vi "Get SplitterPosition.vi"(8 "error in (no error)":errorcluster caption="错误输入（无错误）", 11 "PanelDataNode 输入":refnum<class "PanelDataNode.lvclass"> caption="DNL_LabVIEW Object in") -> (0 "error out":errorcluster caption="错误输出", 2 "SplitterPosition(relative)":dbl, 3 "PanelDataNode 输出":refnum<class "PanelDataNode.lvclass"> caption="DNL_LabVIEW Object out")   [LabVIEW 2016, in "PanelDataNode.lvclass"]
uses:
  PanelDataNode.lvclass
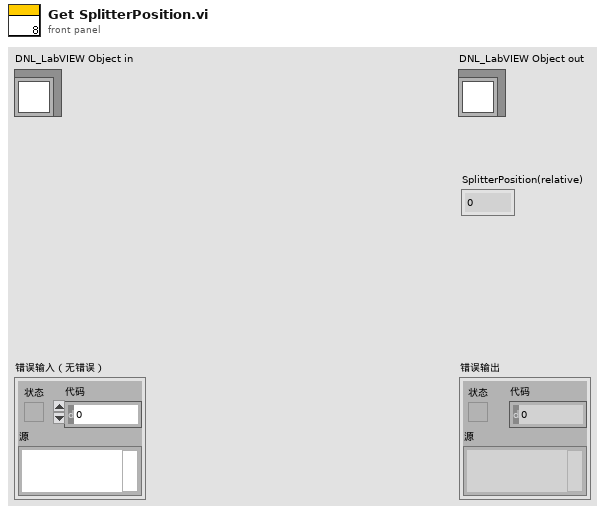
[diagram p1: front panel]
types:
  T1 = typedef "LVBoundsTypeDef.ctl" = cluster{"Width":u32, "Height":u32}
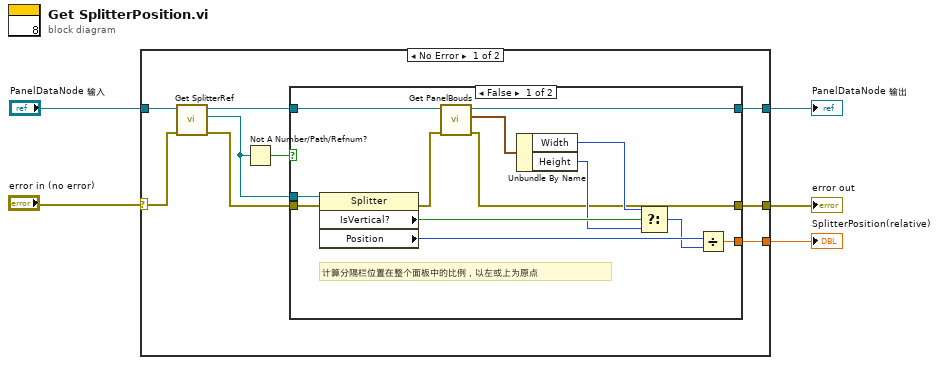
[diagram p0: block diagram]
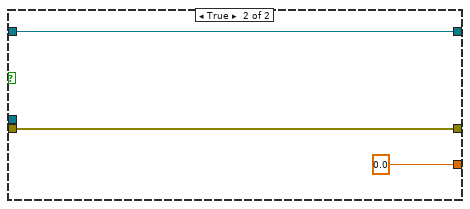
[diagram p2: hidden frame]
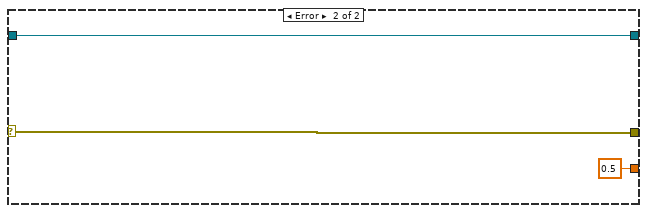
[diagram p3: hidden frame]
diagram:
  n1 = case shown="No Error" "error in (no error)" {
    selector: "error in (no error)" -> [w8 w33]
    tunnel: [w9 w33] -> w4
    tunnel: [w12 w32] -> w2
    tunnel: "PanelDataNode 输入" -> [w14 w32]
    tunnel: [w11 0.5] -> w1
    frame No Error {
      n2 = call "Get SplitterRef.vi"("error in"=w8, "PanelDataNode 输入"=w14) -> ("error out"=w10:errorcluster, "Splitter"=w7:refnum<vi>, "PanelDataNode 输出"=w13:refnum<class "PanelDataNode.lvclass">)  [unwired: 7 in]
      n3 = Not A Number/Path/Refnum?(number/path/refnum=w7) -> (NaN/Path/Refnum?=w6:bool)
      n4 = case shown="False" w6 {
        tunnel: w13 -> [w27 w29]
        tunnel: [w26 w29] -> w12
        tunnel: [w19 0.0] -> w11
        tunnel: w10 -> [w18 w28]
        tunnel: [w16 w28] -> w9
        tunnel: w7 -> [w15 _]
        frame False {
          # "计算分隔栏位置在整个面板中的比例，以左或上为原点"
          n5 = property class="Splitter"(reference=w15, error in=w18) -> (error out=w17:errorcluster, "IsVertical?"=w24:bool, "Position"=w21:i32)  [unwired: 1 out]
          n6 = call "Get PanelBouds.vi"("error in (no error)"=w17, "PanelDataNode 输入"=w27) -> ("error out"=w16:errorcluster, "Bounds"=w25:T1, "PanelDataNode 输出"=w26:refnum<class "PanelDataNode.lvclass">)  [unwired: 7 in]
          n7 = Unbundle By Name(w25) -> ("Width"=w23:u32, "Height"=w22:u32)
          n8 = Select(t=w23, s=w24, f=w22) -> (s? t:f=w20:u32)
          n9 = Divide(x=w21, y=w20) -> (x/y=w19:dbl)
        }
        frame True {
        }
      }
    }
    frame Error {
    }
  }
  "error out" <- w4
  "PanelDataNode 输出" <- w2
  "SplitterPosition(relative)" <- w1
